vi "DSF Configuration Cluster to File.vi"(8 "error in (no error)":errorcluster, 10 "framework configuration":T1, 11 "dsf configuration file path":path) -> (0 "error out":errorcluster, 3 "dsf configuration file path dup":path)   [LabVIEW 2017, in "DSF Core.lvlib"]
uses:
  DSF Core.lvlib
  DSF Configuration API/Public/Controls/DSF Engine Framework Configuration.ctl
  DSF Configuration API/Public/Controls/DSF Engine Plugin Configuration.ctl
  DSF Configuration API/Public/Controls/DSF Timing Info.ctl
  DSF Configuration API/Public/Controls/DSF Engine Plugin Thread Configuration.ctl
  DSF Configuration API/Public/Controls/DSF Settings Info.ctl
  DSF Configuration API/Public/Controls/DSF Engine Transfer Group Configuration.ctl
  DSF Configuration API/Public/Controls/DSF Direction.ctl
  DSF Configuration API/Public/Controls/DSF Engine Transfer Configuration.ctl
  DSF Configuration API/Public/Controls/DSF Byte Order.ctl
  DSF Configuration API/Public/Controls/DSF Engine Channel Configuration.ctl
  DSF Configuration API/Public/Controls/DSF Data Type.ctl
  DSF Configuration API/Public/Controls/DSF Plugin Info.ctl
  DSF Configuration API/Public/Controls/DSF Group Info.ctl
  DSF Configuration API/Public/Controls/DSF Transfer Info.ctl
  DSF Configuration API/Public/Controls/DSF Channel Info.ctl
  DSF Configuration API/Public/Write Item/Write Channel.vi
  DSF Configuration API/Public/Write Item/Write Transfer.vi
  DSF Configuration API/Public/Write Item/Write Group.vi
  DSF Configuration API/Public/Write Item/Write Plugin.vi
  DSF Configuration API/Configuration Session.lvclass
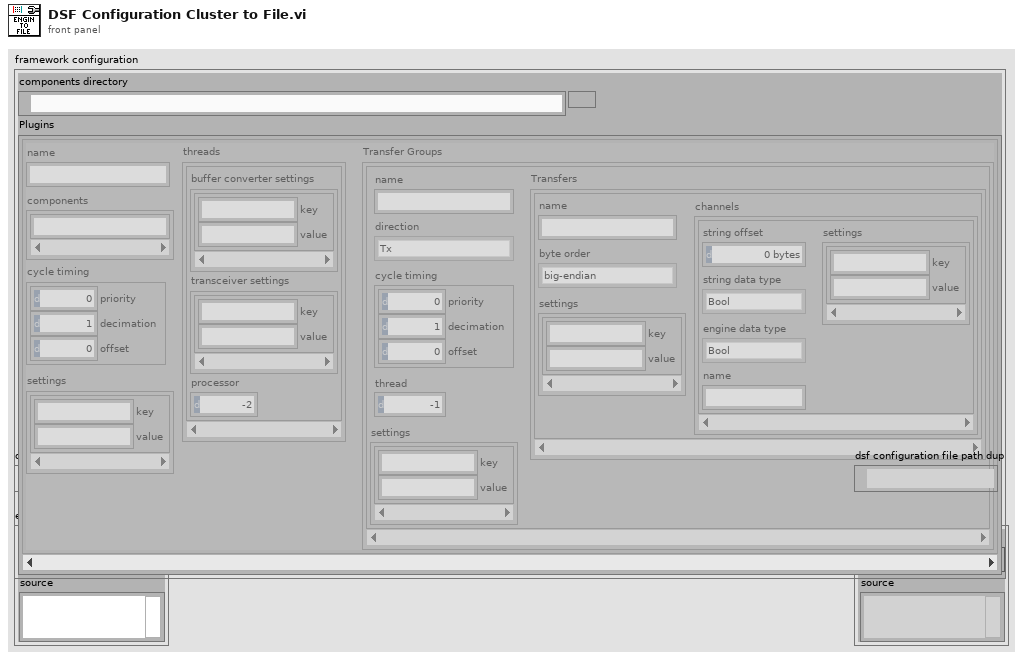
[diagram p1: front panel]
types:
  T1 = typedef "DSF Core.lvlib/DSF Engine Framework Configuration.ctl" = cluster{"components directory":path, "Plugins":T2[]}
  T2 = typedef "DSF Core.lvlib/DSF Engine Plugin Configuration.ctl" = cluster{"name":string, "components":string[], "cycle timing":T3, "threads":T4[], "Transfer Groups":T6[], "settings":T5}
  T3 = typedef "DSF Core.lvlib/DSF Timing Info.ctl" = cluster{"priority":u64, "decimation":u64, "offset":u64}
  T4 = typedef "DSF Core.lvlib/DSF Engine Plugin Thread Configuration.ctl" = cluster{"buffer converter settings":T5, "transceiver settings":T5, "processor":i32}
  T5 = typedef "DSF Core.lvlib/DSF Settings Info.ctl" = cluster{"key":string, "value":string}[]
  T6 = typedef "DSF Core.lvlib/DSF Engine Transfer Group Configuration.ctl" = cluster{"name":string, "direction":T7, "cycle timing":T3, "thread":i32, "settings":T5, "Transfers":T8[]}
  T7 = typedef "DSF Core.lvlib/DSF Direction.ctl" = enum8{"Tx", "Rx"}
  T8 = typedef "DSF Core.lvlib/DSF Engine Transfer Configuration.ctl" = cluster{"name":string, "byte order":T9, "settings":T5, "channels":T10[]}
  T9 = typedef "DSF Core.lvlib/DSF Byte Order.ctl" = enum8{"big-endian", "little-endian"}
  T10 = typedef "DSF Core.lvlib/DSF Engine Channel Configuration.ctl" = cluster{"string offset":u64, "string data type":T11, "engine data type":T11, "name":string, "settings":T5}
  T11 = typedef "DSF Core.lvlib/DSF Data Type.ctl" = enum8{"Bool", "SGL", "DBL", "I8", "I16", "I32", "I64", "U8", "U16", "U32", "U64"}
  T12 = typedef "DSF Core.lvlib/DSF Plugin Info.ctl" = cluster{"components":string[], "timing":T3, "group ids":string[], "settings id":string, "threads":T4[]}
  T13 = typedef "DSF Core.lvlib/DSF Group Info.ctl" = cluster{"direction":T7, "timing":T3, "transfer ids":string[], "settings id":string, "thread":i32}
  T14 = typedef "DSF Core.lvlib/DSF Transfer Info.ctl" = cluster{"byte order":T9, "channel ids":string[], "settings id":string}
  T15 = typedef "DSF Core.lvlib/DSF Channel Info.ctl" = cluster{"string buffer offset":u64, "string data type":T11, "engine data type":T11, "settings id":string}
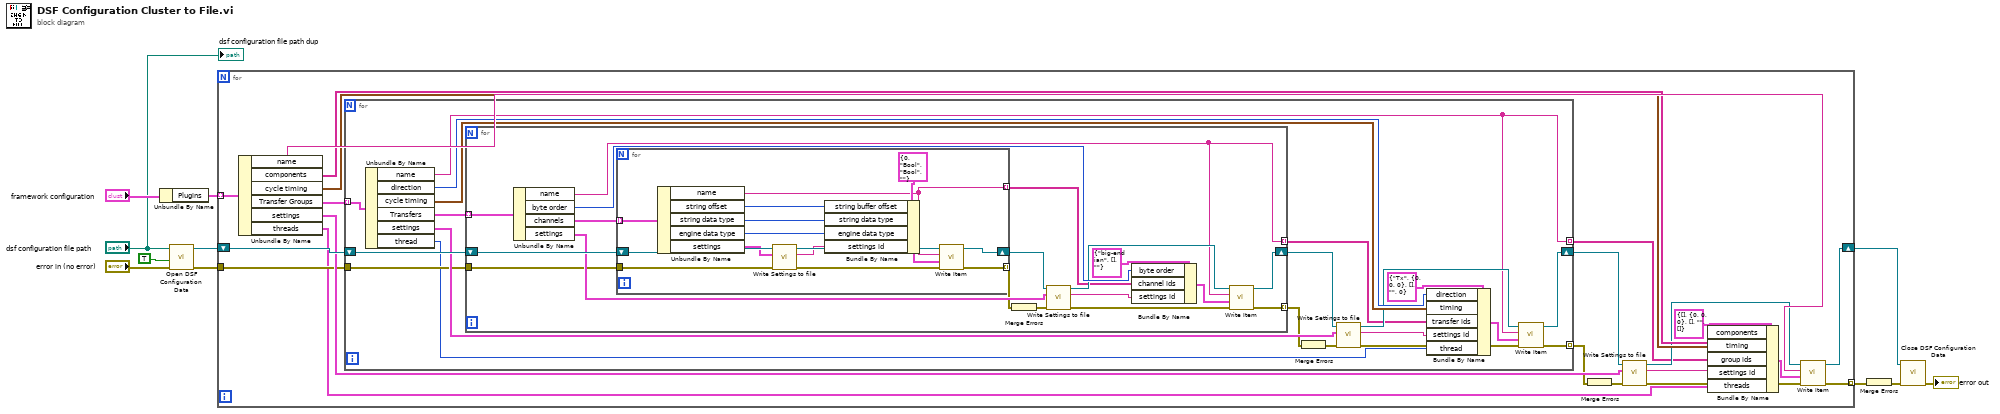
[diagram p0: block diagram]
diagram:
  n1 = Unbundle By Name("framework configuration") -> ("Plugins"=w8:T2[])
  n2 = call "Open DSF Configuration Data.vi"("error in (no error)"="error in (no error)", "replace if found? (F)"=TRUE, "dsf configuration file path"="dsf configuration file path") -> ("error out"=w5:errorcluster, "Configuration Session"=w7:refnum<class "Configuration Session.lvclass">)  [unwired: 4 in, 3 out]
  n3 = for {
    tunnel: w8 -> [w31] mode=indexing
    shift-right: [w23] -> w6
    shift-left: w7 -> [w24]
    tunnel: w5 -> [w17]
    tunnel: [w14] -> w4 mode=indexing
    n4 = Unbundle By Name(w31) -> ("name"=w30:string, "components"=w27:string[], "cycle timing"=w26:T3, "Transfer Groups"=w25:T6[], "settings"=w21:T5, "threads"=w12:T4[])
    n5 = for {
      tunnel: w25 -> [w51] mode=indexing
      shift-right: [w43] -> w19
      shift-left: w24 -> [w45]
      tunnel: [w38] -> w18 mode=indexing
      tunnel: w17 -> [w37]
      tunnel: [w36] -> w16 mode=indexing
      n6 = Unbundle By Name(w51) -> ("name"=w38:string, "direction"=w48:T7, "cycle timing"=w47:T3, "Transfers"=w46:T8[], "settings"=w41:T5, "thread"=w32:i32)
      n7 = for {
        tunnel: w46 -> [w69] mode=indexing
        shift-right: [w62] -> w44
        shift-left: w45 -> [w64]
        tunnel: [w57] -> w39 mode=indexing
        tunnel: w37 -> [w56]
        tunnel: [w53] -> w35 mode=indexing
        n8 = Unbundle By Name(w69) -> ("name"=w57:string, "byte order"=w67:T9, "channels"=w65:T10[], "settings"=w60:T5)
        n9 = for {
          tunnel: w65 -> [w84] mode=indexing
          shift-right: [w81] -> w63
          shift-left: w64 -> [w78]
          tunnel: [w80] -> w58 mode=indexing
          tunnel: w56 -> [w77]
          tunnel: [w79] -> w55 mode=indexing
          n10 = Unbundle By Name(w84) -> ("name"=w80:string, "string offset"=w70:u64, "string data type"=w71:T11, "engine data type"=w72:T11, "settings"=w76:T5)
          n11 = call "Write Settings to file.vi"("error in (no error)"=w77, "settings"=w76, "Configuration Session in"=w78) -> ("error out"=w74:errorcluster, "settings id"=w73:string, "Configuration Session out"=w75:refnum<class "Configuration Session.lvclass">)  [unwired: 6 in]
          n12 = Bundle By Name(cluster=T15 {"string buffer offset"=0, "string data type"=enum."Bool", "engine data type"=enum."Bool", "settings id"=""} ("values"), "string buffer offset"=w70, "string data type"=w71, "engine data type"=w72, "settings id"=w73) -> (w82:T15)
          n13 = call-poly "Write Item.vi"("error in (no error)"=w74, "channel values"=w82, "id"=w80, "Configuration Session in"=w75) -> ("error out"=w79:errorcluster, "Configuration Session out"=w81:refnum<class "Configuration Session.lvclass">)  [unwired: 5 in, 1 out]
        }
        n14 = Merge Errors(w55) -> (w52:errorcluster)
        n15 = call "Write Settings to file.vi"("error in (no error)"=w52, "settings"=w60, "Configuration Session in"=w63) -> ("error out"=w54:errorcluster, "settings id"=w59:string, "Configuration Session out"=w61:refnum<class "Configuration Session.lvclass">)  [unwired: 6 in]
        n16 = Bundle By Name(cluster=T14 {"byte order"=enum."big-endian", "channel ids"=[], "settings id"=""} ("values"), "byte order"=w67, "channel ids"=w58, "settings id"=w59) -> (w66:T14)
        n17 = call-poly "Write Item.vi"("error in (no error)"=w54, "transfer values"=w66, "id"=w57, "Configuration Session in"=w61) -> ("error out"=w53:errorcluster, "Configuration Session out"=w62:refnum<class "Configuration Session.lvclass">)  [unwired: 5 in, 1 out]
      }
      n18 = Merge Errors(w35) -> (w33:errorcluster)
      n19 = call "Write Settings to file.vi"("error in (no error)"=w33, "settings"=w41, "Configuration Session in"=w44) -> ("error out"=w34:errorcluster, "settings id"=w40:string, "Configuration Session out"=w42:refnum<class "Configuration Session.lvclass">)  [unwired: 6 in]
      n20 = Bundle By Name(cluster=T13 {"direction"=enum."Tx", "timing"={"priority"=0, "decimation"=0, "offset"=0}, "transfer ids"=[], "settings id"="", "thread"=0} ("group values"), "direction"=w48, "timing"=w47, "transfer ids"=w39, "settings id"=w40, "thread"=w32) -> (w49:T13)
      n21 = call-poly "Write Item.vi"("error in (no error)"=w34, "group values"=w49, "id"=w38, "Configuration Session in"=w42) -> ("error out"=w36:errorcluster, "Configuration Session out"=w43:refnum<class "Configuration Session.lvclass">)  [unwired: 5 in, 1 out]
    }
    n22 = Merge Errors(w16) -> (w13:errorcluster)
    n23 = call "Write Settings to file.vi"("error in (no error)"=w13, "settings"=w21, "Configuration Session in"=w19) -> ("error out"=w15:errorcluster, "settings id"=w22:string, "Configuration Session out"=w20:refnum<class "Configuration Session.lvclass">)  [unwired: 6 in]
    n24 = Bundle By Name(cluster=T12 {"components"=[], "timing"={"priority"=0, "decimation"=0, "offset"=0}, "group ids"=[], "settings id"="", "threads"=[]} ("plugin values"), "components"=w27, "timing"=w26, "group ids"=w18, "settings id"=w22, "threads"=w12) -> (w28:T12)
    n25 = call-poly "Write Item.vi"("error in (no error)"=w15, "plugin values"=w28, "id"=w30, "Configuration Session in"=w20) -> ("error out"=w14:errorcluster, "Configuration Session out"=w23:refnum<class "Configuration Session.lvclass">)  [unwired: 5 in, 1 out]
  }
  n26 = Merge Errors(w4) -> (w2:errorcluster)
  n27 = call "Close DSF Configuration Data.vi"("error in (no error)"=w2, "Configuration Session"=w6) -> ("error out"=→"error out":errorcluster)  [unwired: 8 in, 1 out]
  "dsf configuration file path dup" <- "dsf configuration file path"
